vi "Add Database to SysDef.vi"(8 "error in":errorcluster, 10 "DB Alias":string="Diagnostics_Addon_Temp_DB", 11 "Item Ref in":T1 format="%.0x") -> (0 "error out":errorcluster, 3 "Item Ref out":T1 format="%.0x")   [LabVIEW 2023, in "J1939 Addon System Explorer.lvlib"]
uses:
  J1939 Addon System Explorer.lvlib
  <vilib>/NI VeriStand/Custom Device API/Custom Device Item Ref.ctl
  <vilib>/NI VeriStand/Custom Device Tools/Custom Device Utility Library/NI VeriStand - Search for Item by GUID.vi
  <vilib>/NI VeriStand/Custom Device Tools/Custom Device Utility Library/NI VeriStand - Search for Item by Name.vi
  <vilib>/NI VeriStand/Custom Device API/Set Item Property (String).vi
  <vilib>/NI VeriStand/Custom Device Tools/Custom Device Utility Library/Custom Device Utility Library.lvlib
  <vilib>/NI VeriStand/Custom Device API/Custom Device API.lvlib
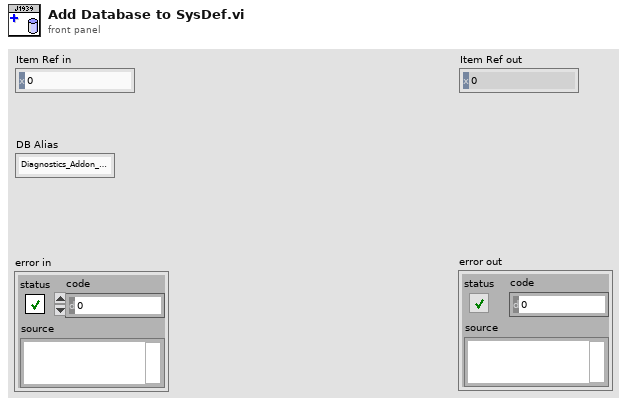
[diagram p1: front panel]
types:
  T1 = typedef "Custom Device API.lvlib/Custom Device Item Ref.ctl" = u64
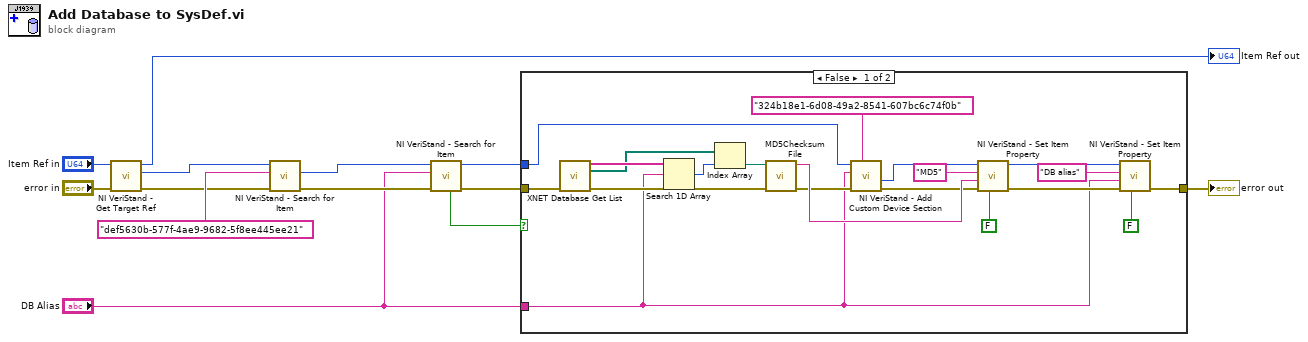
[diagram p0: block diagram]
diagram:
  n1 = call <vilib>:"NI VeriStand - Get Target Ref.vi"("error in"="error in", "Item Ref in"="Item Ref in") -> ("error out"=w10:errorcluster, "Target Ref"=w9:T1, "Item Ref out"=→"Item Ref out":T1)  [unwired: 6 in, 1 out]
  n2 = call-poly <vilib>:"NI VeriStand - Search for Item.vi"("error in"=w10, "Item GUID"="def5630b-577f-4ae9-9682-5f8ee445ee21" ("string"), "Section Ref in"=w9) -> ("error out"=w11:errorcluster, "Item Ref"=w12:T1)  [unwired: 5 in, 2 out]
  n3 = call-poly <vilib>:"NI VeriStand - Search for Item.vi"("error in"=w11, "Item Name"="DB Alias", "Section Ref in"=w12) -> ("error out"=w8:errorcluster, "Section Ref out"=w7:T1, "Found"=w6:bool)  [unwired: 5 in, 1 out]
  n4 = case shown="False" w6 {
    tunnel: [w22 w34] -> w5
    tunnel: w8 -> [w20 w34]
    tunnel: w7 -> [w21 _]
    tunnel: "DB Alias" -> [w17 _]
    frame False {
      n5 = call <vilib>:"XNET Database Get List.vi"("error in (no error)"=w20) -> ("array of alias"=w18:string[], "array of filepath"=w15:path[], "error out"=w19:errorcluster)  [unwired: 12 in]
      n6 = Search 1D Array(1D array=w18, element=w17) -> (index of element=w16:i32)  [unwired: 1 in]
      n7 = Index Array(array=w15, index=w16) -> (element=w14:path)
      n8 = call <vilib>:"MD5Checksum File.vi"("error in (no error)"=w19, "Path"=w14) -> ("error out"=w32:errorcluster, "MD5 message-digest"=w33:string)  [unwired: 8 in]
      n9 = call <vilib>:"NI VeriStand - Add Custom Device Section.vi"("GUID (Default Section)"="324b18e1-6d08-49a2-8541-607bc6c74f0b", "error in (no error)"=w32, "Section Name"=w17, "Parent Ref in"=w21) -> ("error out"=w26:errorcluster, "Section Ptr"=w25:T1)  [unwired: 4 in, 2 out]
      n10 = call-poly <vilib>:"NI VeriStand - Set Item Property.vi"("Binary String (T)"=FALSE, "error in (no error)"=w26, "Value"=w33, "Property Name"="MD5", "Item Ref in"=w25) -> ("error out"=w27:errorcluster, "Item Ref out"=w28:T1)  [unwired: 4 in, 1 out]
      n11 = call-poly <vilib>:"NI VeriStand - Set Item Property.vi"("Binary String (T)"=FALSE, "error in (no error)"=w27, "Value"=w17, "Property Name"="DB alias", "Item Ref in"=w28) -> ("error out"=w22:errorcluster)  [unwired: 4 in, 2 out]
    }
    frame True {
    }
  }
  "error out" <- w5
